vi "ModifyXmitParams.vi"(10 "TimeShifts":T1(array[cluster]), 11 "Recip Table":i16[][](array[numeric])) -> (2 "New Time Shift":T1(array[cluster]), 3 "New Recip Table":i16[][](array[numeric]))   [LabVIEW 2022 SP3]
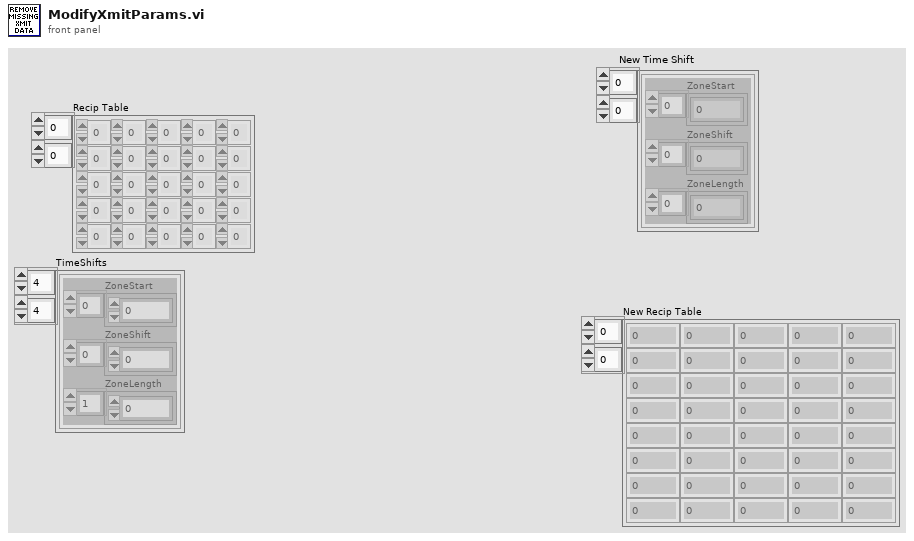
[diagram p1: front panel]
types:
  T1 = cluster{"ZoneStart":sgl[], "ZoneShift":sgl[], "ZoneLength":sgl[]}[][]
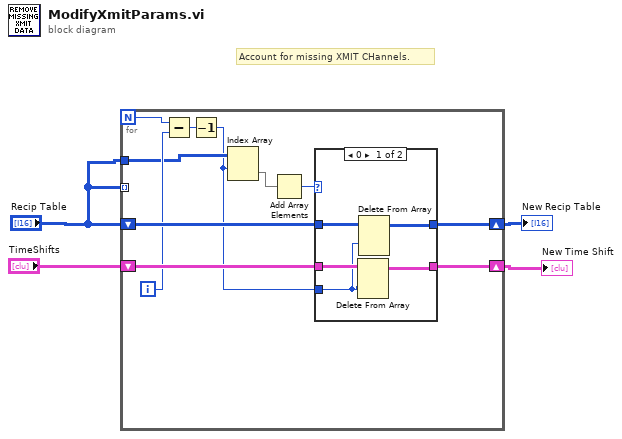
[diagram p0: block diagram]
diagram:
  # "Account for missing XMIT CHannels."
  n1 = for {
    N -> [w6]
    tunnel: "Recip Table" -> [_] mode=indexing
    shift-right: [w12] -> w4
    shift-left: "Recip Table" -> [w14]
    shift-right: [w11] -> w3
    shift-left: "TimeShifts" -> [w15]
    tunnel: "Recip Table" -> [w8]
    i -> [w10]
    n2 = Subtract(x=w6, y=w10) -> (x-y=w9:i32)
    n3 = Decrement(x=w9) -> (x-1=w5:i32)
    n4 = Index Array(array=w8, index (row)=w5) -> (element=w7:i16[])  [unwired: 1 in]
    n5 = Add Array Elements(numeric array=w7) -> (sum=w13:i16)
    n6 = case shown="0" w13 {
      tunnel: w15 -> [w19 w21]
      tunnel: w14 -> [w20 w22]
      tunnel: w5 -> [w16 _]
      tunnel: [w18 w22] -> w12
      tunnel: [w17 w21] -> w11
      frame 0 {
        n7 = Delete From Array(array=w19, index (row)=w16) -> (array with subset deleted=w17:T1)  [unwired: 2 in, 1 out]
        n8 = Delete From Array(array=w20, index (row)=w16) -> (array with subset deleted=w18:i16[][])  [unwired: 2 in, 1 out]
      }
      frame 1, Default {
      }
    }
  }
  "New Recip Table" <- w4
  "New Time Shift" <- w3
